vi "reconstruct single image for saving channel 2.vi"(6 "bidirection?":bool=TRUE, 7 "x fly back pixel":u16, 8 "PXI channel":T1={"Vertical Range (V)"=1.0, "Min Sample Rate"=2208791.906743315, "# of Channels"=1, "Min Record Length"=560, "Number Of Records"=10000, "Trigger Position(%)"=0.0, "act Record Length"=1000, "trigger source"="VAL_EXTERNAL", "PMT2 # of Channels"=1} {"PMT2 # of Channels" min=1 max=8 step=1; "act Record Length" min=0 max=100000 step=1 format="%#.3g"; "Trigger Position(%)" min=0.0 max=100.0 format="%#.3p"; "Number Of Records" min=0 max=1000000 step=1 format="%#.3g"; "Min Record Length" min=0 max=10000 step=1; "# of Channels" min=1 max=8 step=1; "Min Sample Rate" min=0.0 max=100000000.0 format="%#.3p"; "Vertical Range (V)" min=0.0 max=10.0 format="%#.3g"}, 9 "advanced params":T4={"x flyback time(%)"=40.0, "signal offset"=0, "frame time(s)"=0.0, "fetch # per frame"=1, "galvo sampling rate"=0} {"galvo sampling rate" max=100 step=1 format="%#.3g"; "fetch # per frame" max=100 step=1 format="%#.3g"; "frame time(s)" min=0.0 max=10000.0 format="%#.3g"; "signal offset" max=200 format="%#.3g"; "x flyback time(%)" min=0.0 max=200.0 format="%#.3g"}, 10 "basic params":T3={"X pixel #"=200, "X pixel size(um)"=1.0, "Y pixel #"=200, "Y pixel size(um)"=10.0, "line rate(Hz)"=1.0, "stage scan?"=FALSE} {"line rate(Hz)" min=1.0 max=2000.0 format="%#.3g"; "X pixel size(um)" min=0.0 max=10.0 format="%#.3g"; "X pixel #" min=2 max=20480 step=2 format="%#.3g"; "Y pixel size(um)" min=0.0 max=10.0 format="%#.3g"; "Y pixel #" min=2 max=204800 step=2 format="%#.3g"}, 11 "raw data":i16[][](array[numeric])) -> (3 "images":i16[][][](array[numeric]))   [LabVIEW 2015]
uses:
  type def/advanced params.ctl
  type def/basic params.ctl
  type def/PXI control.ctl
  <instrlib>/niScope/Controls/niScope trigger source digital.ctl
panel:
  in  "index (page)":i32
  out "final image":i16[][](graph)
  out "recombine image":i16[][](graph)
  out "backward direction":i16[][](graph)
  out "forward directon":i16[][](graph)
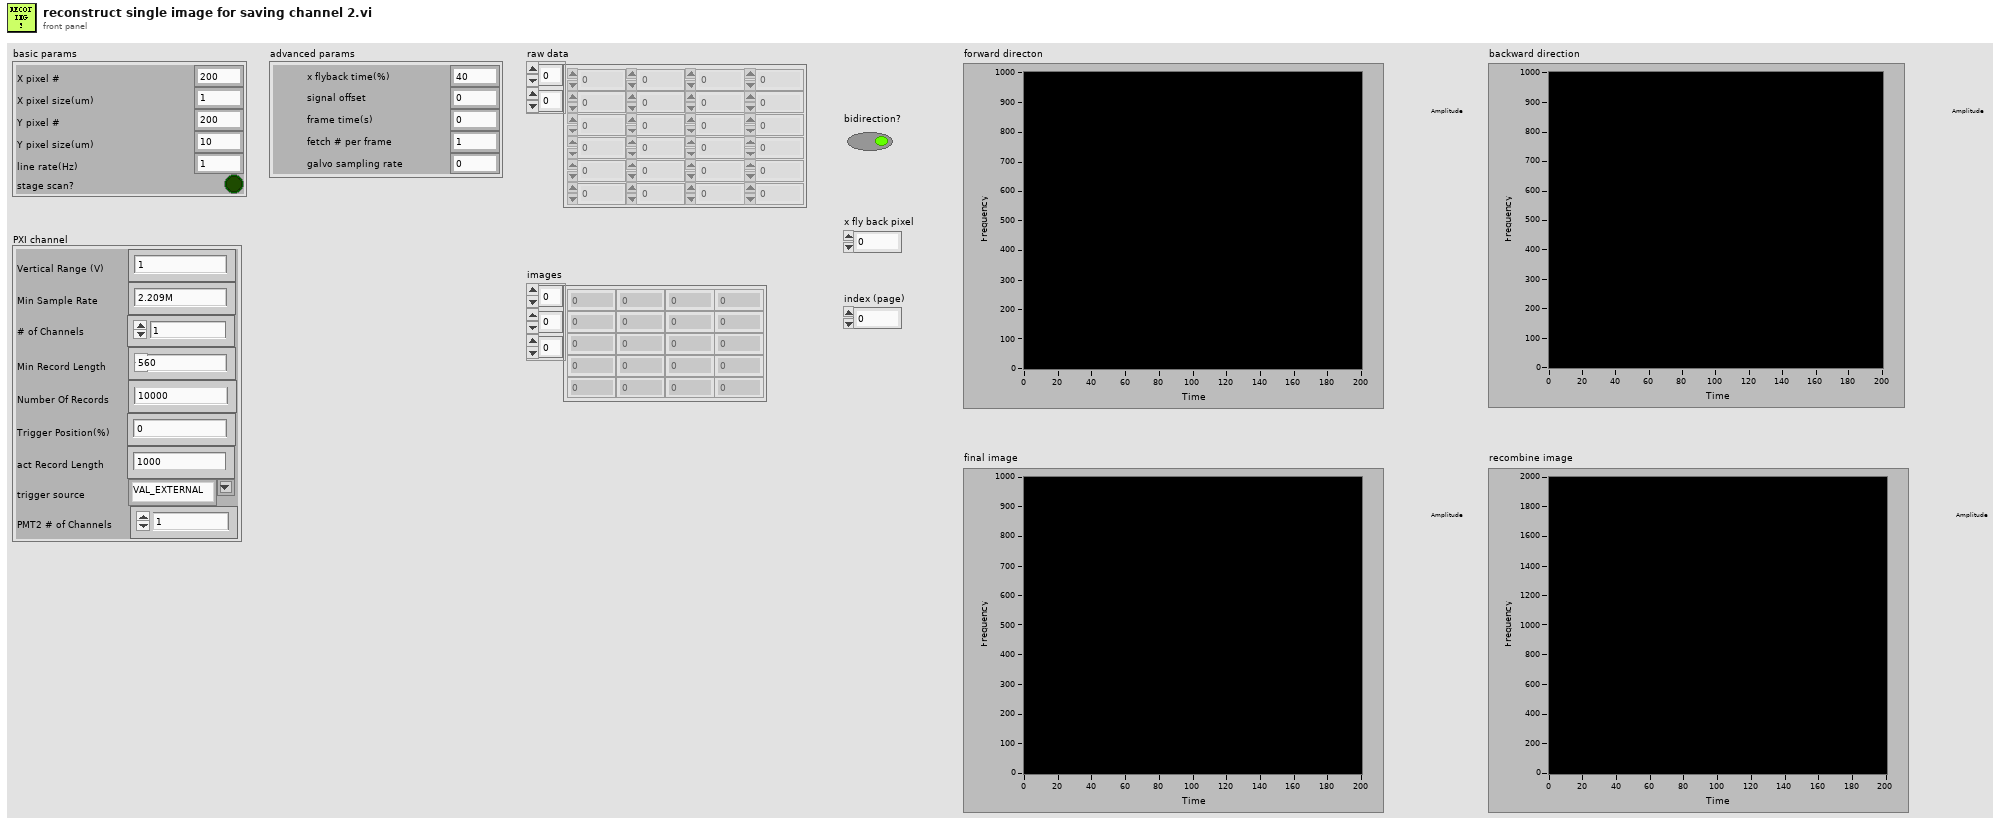
[diagram p1: front panel]
types:
  T1 = typedef "PXI control.ctl" = cluster{"Vertical Range (V)":dbl, "Min Sample Rate":dbl, "# of Channels":u8, "Min Record Length":i32, "Number Of Records":i32, "Trigger Position(%)":dbl, "act Record Length":i32, "trigger source":T2, "PMT2 # of Channels":u8}
  T2 = typedef "niScope trigger source digital.ctl" = string
  T3 = typedef "basic params.ctl" = cluster{"X pixel #":u32, "X pixel size(um)":dbl, "Y pixel #":u32, "Y pixel size(um)":dbl, "line rate(Hz)":dbl, "stage scan?":bool}
  T4 = typedef "advanced params.ctl" = cluster{"x flyback time(%)":dbl, "signal offset":u16, "frame time(s)":dbl, "fetch # per frame":u16, "galvo sampling rate":u32}
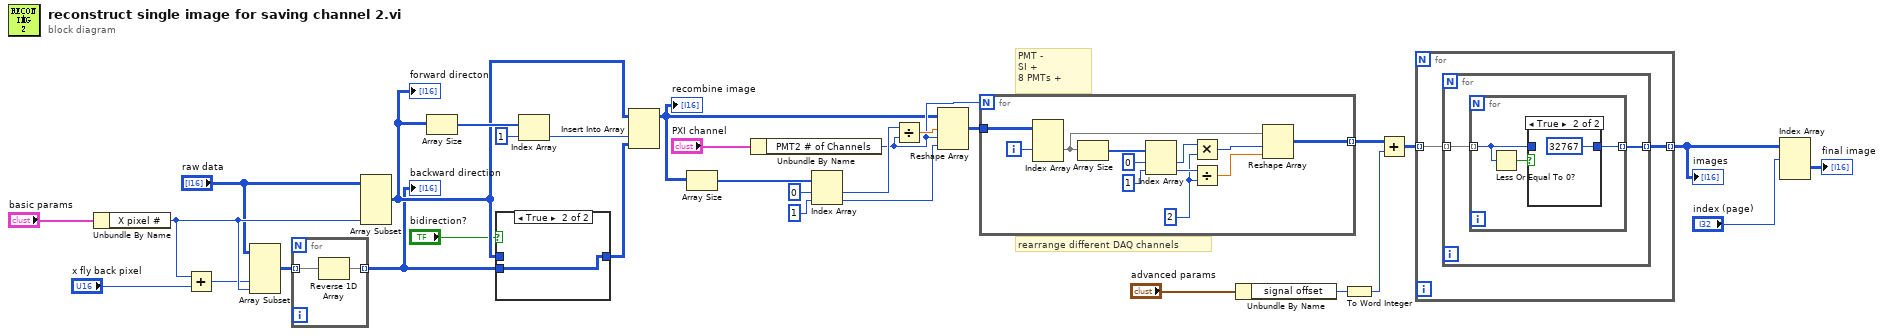
[diagram p0: block diagram]
diagram:
  # "PMT -\nSI +\n8 PMTs +"
  # "rearrange different DAQ channels"
  n1 = Unbundle By Name("basic params") -> ("X pixel #"=w30:u32)
  n2 = Add(x=w30, y="x fly back pixel") -> (x+y=w29:u32)
  n3 = Array Subset(array="raw data", index (col)=w29, length (col)=w30) -> (w28:i16[][])  [unwired: 2 in]
  n4 = for {
    tunnel: w28 -> [w33] mode=indexing
    tunnel: [w32] -> w9 mode=indexing
    n5 = Reverse 1D Array(array=w33) -> (reversed array=w32:i16[])
  }
  "backward direction" <- w9
  n6 = Array Subset(array="raw data", length (col)=w30) -> (w11:i16[][])  [unwired: 3 in]
  "forward directon" <- w11
  n7 = Array Size(array=w11) -> (size(s)=w27:i32[])
  n8 = case shown="True" "bidirection?" {
    tunnel: w11 -> [w34 _]
    tunnel: [w34 w35] -> w10
    tunnel: w9 -> [_ w35]
    frame False {
    }
    frame True {
    }
  }
  n9 = Index Array(array=w27, index=1) -> (element=w25:i32)
  n10 = Insert Into Array(array=w11, index (col)=w25, new element=w10) -> (w15:i16[][])  [unwired: 1 in]
  "recombine image" <- w15
  n11 = Array Size(array=w15) -> (size(s)=w18:i32[])
  n12 = Unbundle By Name("PXI channel") -> ("PMT2 # of Channels"=w17:u8)
  n13 = Index Array(array=w18, index #1=0 ("index"), index #2=1 ("index")) -> (element #1=w22:i32, element #2=w19:i32)
  n14 = Divide(x=w22, y=w17) -> (x/y=w24:dbl)
  n15 = Reshape Array(w15, w24, w17, w19) -> (w23:i16[][][])
  n16 = for {
    N: w17 -> [_]
    tunnel: w23 -> [w47]
    tunnel: [w37] -> w4 mode=indexing
    i -> [w46]
    w40 = 2 ("y")
    n17 = Index Array(array=w47, index (dim 1)=w46) -> (element=w36:i16[][])  [unwired: 2 in]
    n18 = Array Size(array=w36) -> (size(s)=w44:i32[])
    n19 = Index Array(array=w44, index #1=0 ("index (row)"), index #2=1 ("disabled index (col)")) -> (element #1=w39:i32, element #2=w42:i32)
    n20 = Multiply(x=w39, y=w40) -> (x*y=w38:i32)
    n21 = Divide(x=w42, y=w40) -> (x/y=w41:dbl)
    n22 = Reshape Array(w36, w38, w41) -> (w37:i16[][])
  }
  n23 = Unbundle By Name("advanced params") -> ("signal offset"=w16:u16)
  n24 = To Word Integer(number=w16) -> (16bit integer=w3:i16)
  n25 = Add(x=w4, y=w3) -> (x+y=w2:i16[][][])
  n26 = for {
    tunnel: w2 -> [w49] mode=indexing
    tunnel: [w48] -> w1 mode=indexing
    n27 = for {
      tunnel: w49 -> [w51] mode=indexing
      tunnel: [w50] -> w48 mode=indexing
      n28 = for {
        tunnel: w51 -> [w53] mode=indexing
        tunnel: [w54] -> w50 mode=indexing
        n29 = Less Or Equal To 0?(x=w53) -> (x <= 0?=w52:bool)
        n30 = case shown="True" w52 {
          tunnel: [w55 i16 32767 ("x")] -> w54
          tunnel: w53 -> [w55 _]
          frame False {
          }
          frame True {
          }
        }
      }
    }
  }
  "images" <- w1
  n31 = Index Array(array=w1, index (dim 0)="index (page)") -> (element=→"final image":i16[][])  [unwired: 2 in]
